vi "GT_Reset.vi"(1 "rtn_In":cluster{"rtn":i16, "Func":string}) -> (0 "rtn_Out":cluster{"rtn":i16, "Func":string})   [LabVIEW 2014]
uses:
  VC6/gts.dll
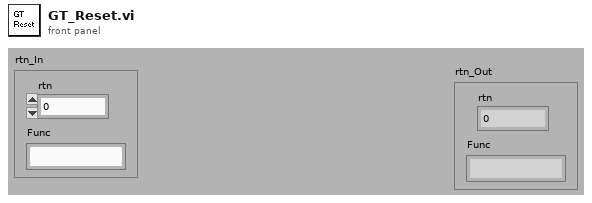
[diagram p1: front panel]
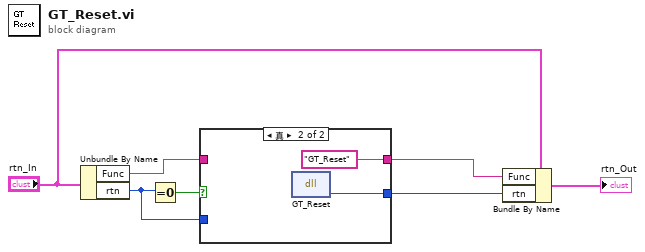
[diagram p0: block diagram]
diagram:
  n1 = Unbundle By Name("rtn_In") -> ("Func"=w3:string, "rtn"=w2:i16)
  n2 = Equal To 0?(x=w2) -> (x = 0?=w7:bool)
  n3 = case shown="真" w7 {
    tunnel: [w8 w11] -> w5
    tunnel: [w9 "GT_Reset" ("Func")] -> w4
    tunnel: w3 -> [w9 _]
    tunnel: w2 -> [w8 _]
    frame False {
    }
    frame True {
      n4 = dll-call lib="PTH2Fabs DNewGTS AC-800LWin7版源程序-20170926gts85VC6gts.dll" fn="GT_Reset"() -> ("rtn"=w11:i16)  [unwired: 3 in, 2 out]
    }
  }
  n5 = Bundle By Name(cluster="rtn_In", "Func"=w4, "rtn"=w5) -> (→"rtn_Out":cluster{"rtn":i16, "Func":string})
